vi "Gateway_Close.vi"(8 "error in (no error)":errorcluster, 11 "GatewayClass in":refnum<class "GatewayClass.lvclass">) -> (0 "error out":errorcluster, 3 "GatewayClass out":refnum<class "GatewayClass.lvclass">)   [LabVIEW 2018, in "GatewayClass.lvclass"]
uses:
  GatewayClass.lvclass
  GatewayClass.lvclass/GatewayClass.ctl
  DataPacker/Utilities/SSH_TUNNEL.lvclass
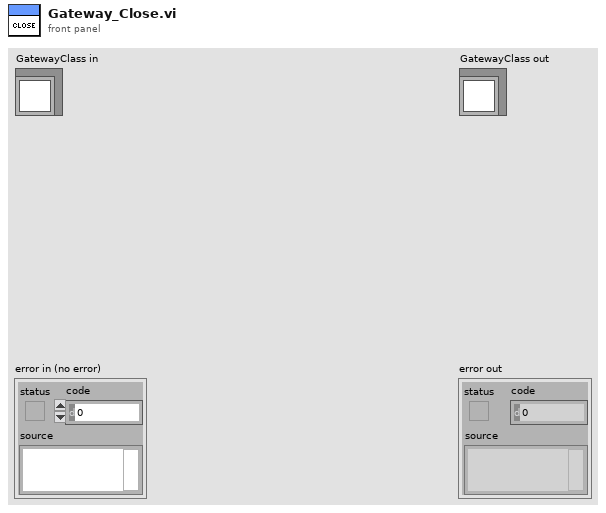
[diagram p1: front panel]
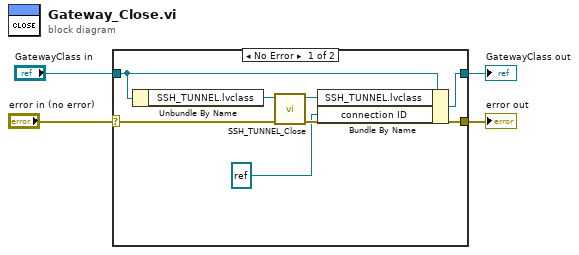
[diagram p0: block diagram]
diagram:
  n1 = case shown="No Error" "error in (no error)" {
    selector: "error in (no error)" -> [w11 w13]
    tunnel: [w9 w13] -> w3
    tunnel: [w6 w12] -> w1
    tunnel: "GatewayClass in" -> [w8 w12]
    frame No Error {
      n2 = Unbundle By Name(w8) -> ("SSH_TUNNEL.lvclass"=w10:refnum<class "SSH_TUNNEL.lvclass">)
      n3 = call "SSH_TUNNEL_Close.vi"("error in (no error)"=w11, "SSH_TUNNEL in"=w10) -> ("error out"=w9:errorcluster, "SSH_TUNNEL out"=w7:refnum<class "SSH_TUNNEL.lvclass">)  [unwired: 8 in]
      n4 = Bundle By Name(cluster=w8, "SSH_TUNNEL.lvclass"=w7, "connection ID"=refnum<k5> refnum) -> (w6:refnum<class "GatewayClass.lvclass">)
    }
    frame Error {
    }
  }
  "error out" <- w3
  "GatewayClass out" <- w1
